vi "四点权值_白子.vi"(0 "3位置行":dbl, 1 "2位置行":dbl, 2 "1位置行":dbl, 3 "当前棋盘状态":i32[][](array[numeric]), 5 "4位置行":dbl, 9 "1位置列":i8, 11 "2位置列":i8, 12 "3位置列":i8, 13 "4位置列":i8) -> (4 "白子四位置权值":i32, 6 "有2个白子?或白子加无子?":bool, 8 "第1个是白子？":bool, 10 "3个白子?":bool, 14 "第一个位置为空？":bool, 15 "3个白子？或2个白子加无子":bool)   [LabVIEW 2018]
panel:
  out "第四位在框内？":bool
  out "第三位在框内？":bool
  out "第二位在框内？":bool
  out "第一位在框内？":bool
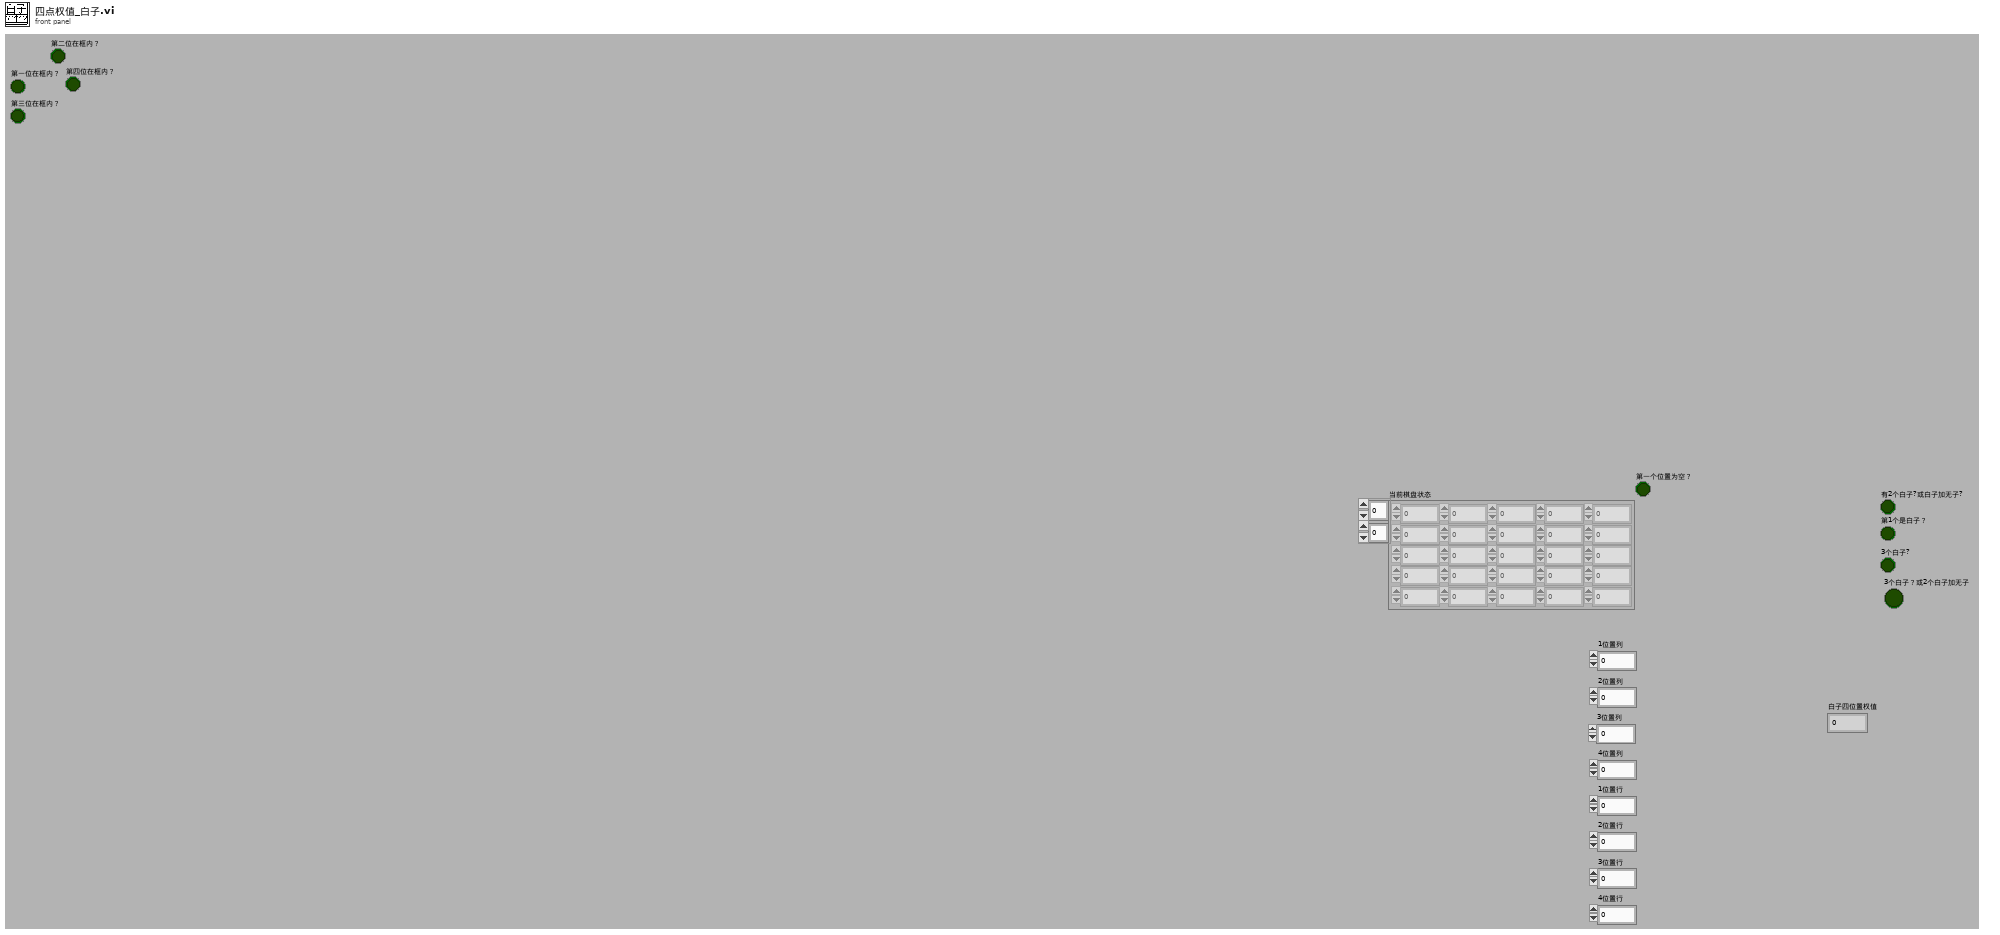
[diagram p1: front panel]
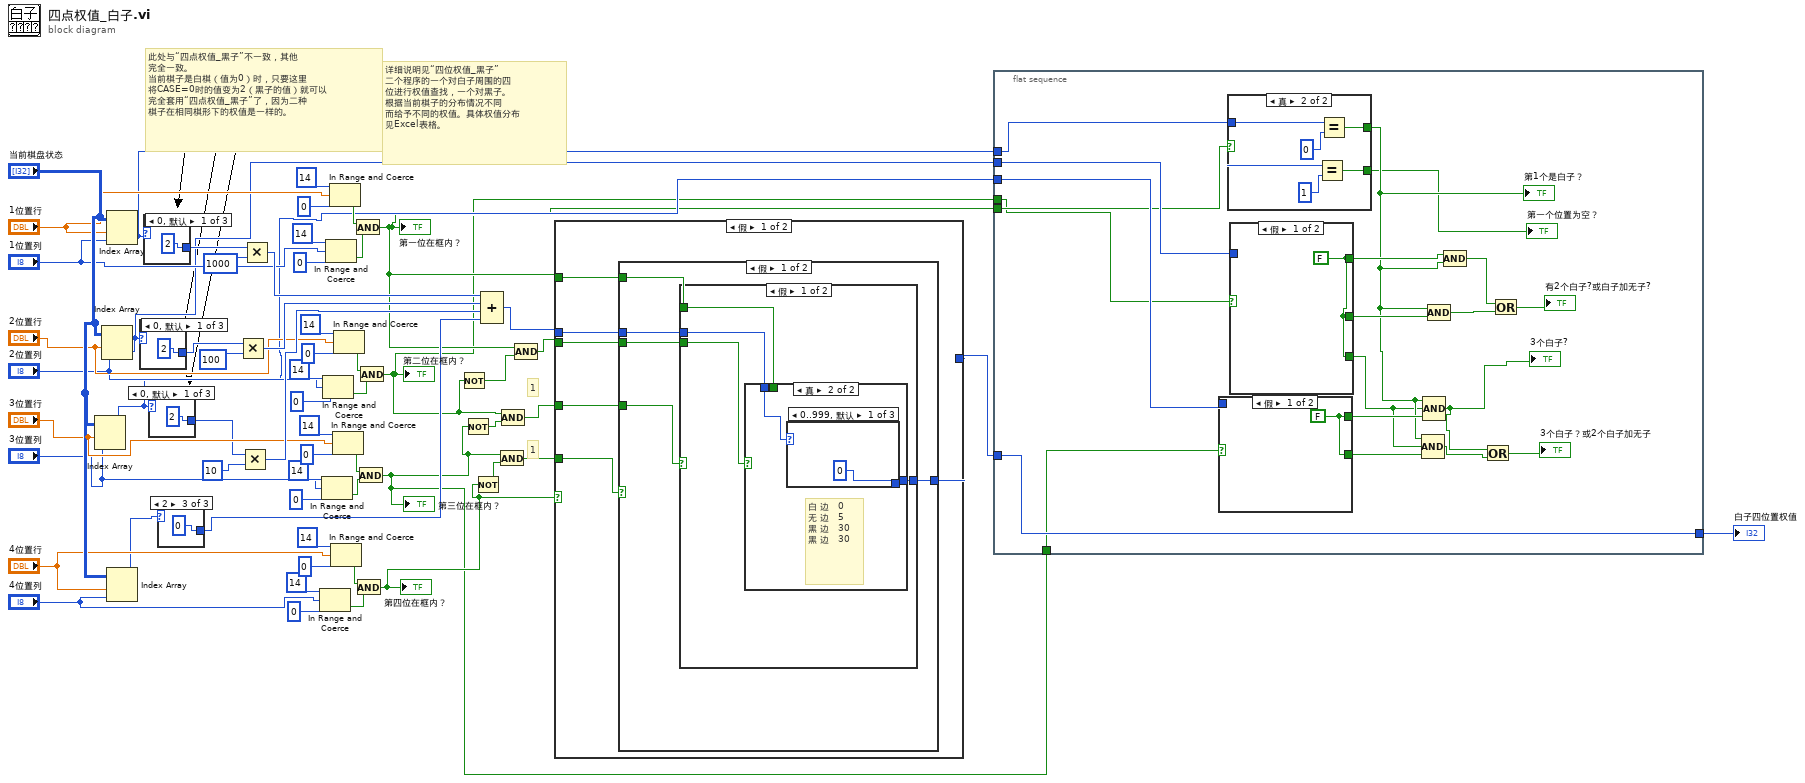
[diagram p0: block diagram]
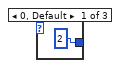
[diagram p2: hidden frame]
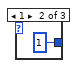
[diagram p3: hidden frame]
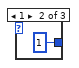
[diagram p4: hidden frame]
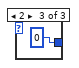
[diagram p5: hidden frame]
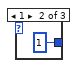
[diagram p6: hidden frame]
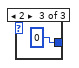
[diagram p7: hidden frame]
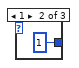
[diagram p8: hidden frame]
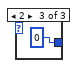
[diagram p9: hidden frame]
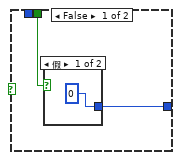
[diagram p10: hidden frame]
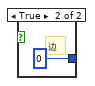
[diagram p11: hidden frame]
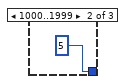
[diagram p12: hidden frame]
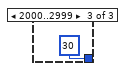
[diagram p13: hidden frame]
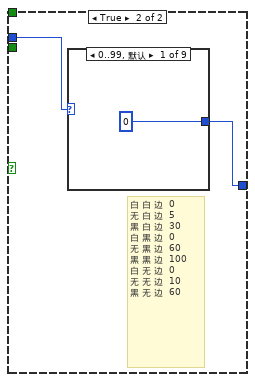
[diagram p14: hidden frame]
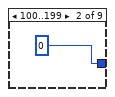
[diagram p15: hidden frame]
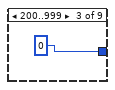
[diagram p16: hidden frame]
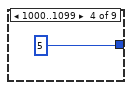
[diagram p17: hidden frame]
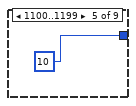
[diagram p18: hidden frame]
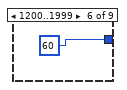
[diagram p19: hidden frame]
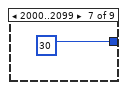
[diagram p20: hidden frame]
diagram:
  # "此处与“四点权值_黑子”不一致，其他\n完全一致。\n当前棋子是白棋（值为0）时，只要这里\n将CASE=0时的值变为2（黑子的值）就可以\n完全套用“四点权值_黑子”了，因为二种\n棋子在相同棋形下的权值是一样的。"
  # "详细说明见“四位权值_黑子”\n二个程序的一个对白子周围的四\n位进行权值查找，一个对黑子。\n根据当前棋子的分布情况不同\n而给予不同的权值。具体权值分布\n见Excel表格。"
  # "1"
  # "1"
  n1 = Index Array(array="当前棋盘状态", index (row)="3位置行", index (col)="3位置列") -> (element=w4:i32)
  n2 = Index Array(array="当前棋盘状态", index (row)="2位置行", index (col)="2位置列") -> (element=w5:i32)
  n3 = Index Array(array="当前棋盘状态", index (row)="1位置行", index (col)="1位置列") -> (element=w6:i32)
  n4 = Index Array(array="当前棋盘状态", index (row)="4位置行", index (col)="4位置列") -> (element=w8:i32)
  n5 = case shown="0, 默认" w5 {
    tunnel: [2 1 0] -> w10
    frame 0, Default {
    }
    frame 1 {
    }
    frame 2 {
    }
  }
  n6 = case shown="0, 默认" w6 {
    tunnel: [2 1 0] -> w11
    frame 0, Default {
    }
    frame 1 {
    }
    frame 2 {
    }
  }
  n7 = case shown="0, 默认" w4 {
    tunnel: [2 1 0] -> w9
    frame 0, Default {
    }
    frame 1 {
    }
    frame 2 {
    }
  }
  n8 = case shown="2" w8 {
    tunnel: [2 1 0] -> w7
    frame 0, Default {
    }
    frame 1 {
    }
    frame 2 {
    }
  }
  n9 = Multiply(x=w10, y=100) -> (x*y=w25:i32)
  n10 = Multiply(x=w9, y=10) -> (x*y=w24:i32)
  n11 = Multiply(x=w11, y=1000) -> (x*y=w26:i32)
  n12 = In Range and Coerce(upper limit=14, x="4位置列", lower limit=0) -> (In Range?=w40:bool)  [unwired: 1 out]
  n13 = In Range and Coerce(upper limit=14, x="3位置列", lower limit=0) -> (In Range?=w34:bool)  [unwired: 1 out]
  n14 = In Range and Coerce(upper limit=14, x="2位置列", lower limit=0) -> (In Range?=w54:bool)  [unwired: 1 out]
  n15 = In Range and Coerce(upper limit=14, x="1位置列", lower limit=0) -> (In Range?=w55:bool)  [unwired: 1 out]
  n16 = In Range and Coerce(upper limit=14, x="1位置行", lower limit=0) -> (In Range?=w56:bool)  [unwired: 1 out]
  n17 = In Range and Coerce(upper limit=14, x="4位置行", lower limit=0) -> (In Range?=w41:bool)  [unwired: 1 out]
  n18 = In Range and Coerce(upper limit=14, x="3位置行", lower limit=0) -> (In Range?=w35:bool)  [unwired: 1 out]
  n19 = In Range and Coerce(upper limit=14, x="2位置行", lower limit=0) -> (In Range?=w53:bool)  [unwired: 1 out]
  n20 = And(x=w56, y=w55) -> (x .and. y?=w3:bool)
  "第一位在框内？" <- w3
  n21 = And(x=w41, y=w40) -> (x .and. y?=w32:bool)
  "第四位在框内？" <- w32
  n22 = And(x=w35, y=w34) -> (x .and. y?=w1:bool)
  "第三位在框内？" <- w1
  n23 = And(x=w53, y=w54) -> (x .and. y?=w2:bool)
  "第二位在框内？" <- w2
  n24 = Not(x=w2) -> (.not. x?=w30:bool)
  n25 = Not(x=w1) -> (.not. x?=w28:bool)
  n26 = Not(x=w32) -> (.not. x?=w29:bool)
  n27 = Compound Arithmetic op=ADD(w26, w25, w24, w7) -> (w23:i32)
  n28 = And(x=w1, y=w29) -> (x .and. y?=w33:bool)
  n29 = Compound Arithmetic op=AND(w2, w28) -> (w31:bool)
  n30 = Compound Arithmetic op=AND(w3, w30) -> (w27:bool)
  n31 = case shown="假" w32 {
    tunnel: [w74 w126] -> w12
    tunnel: w33 -> [w78 _]
    tunnel: w31 -> [w77 _]
    tunnel: w27 -> [w76 _]
    tunnel: w3 -> [w75 _]
    tunnel: w23 -> [w73 w127]
    frame False {
      n32 = case shown="假" w78 {
        tunnel: w77 -> [w83 _]
        tunnel: w76 -> [w82 _]
        tunnel: w75 -> [w81 _]
        tunnel: [w80 w108] -> w74
        tunnel: w73 -> [w79 w109]
        frame False {
          n33 = case shown="假" w83 {
            tunnel: w82 -> [w87 _]
            tunnel: w81 -> [w86 _]
            tunnel: [w85 w97] -> w80
            tunnel: w79 -> [w84 w98]
            frame False {
              n34 = case shown="真" w87 {
                tunnel: w86 -> [w89 _]
                tunnel: [w88 w92] -> w85
                tunnel: w84 -> [_ w93]
                frame False {
                  n35 = case shown="假" w89 {
                    tunnel: [0 0] -> w88
                    frame False {
                    }
                    frame True {
                      # "边"
                    }
                  }
                }
                frame True {
                  # "白\t边\t\t\t0\n无\t边\t\t\t5\n黑\t边\t\t\t30\n黑\t边\t\t\t30"
                  n36 = case shown="0..999, 默认" w93 {
                    tunnel: [0 5 30] -> w92
                    frame 0..999, Default {
                    }
                    frame 1000..1999 {
                    }
                    frame 2000..2999 {
                    }
                  }
                }
              }
            }
            frame True {
              # "白\t白\t边\t\t0\n无\t白\t边\t\t5\n黑\t白\t边\t\t30\n白\t黑\t边\t\t0\n无\t黑\t边\t\t60\n黑\t黑\t边\t\t100\n白\t无\t边\t\t0\n无\t无\t边\t\t10\n黑\t无\t边\t\t60"
              n37 = case shown="0..99, 默认" w98 {
                tunnel: [0 0 0 5 10 60 30 60 100] -> w97
                frame 0..99, Default {
                }
                frame 100..199 {
                }
                frame 200..999 {
                }
                frame 1000..1099 {
                }
                frame 1100..1199 {
                }
                frame 1200..1999 {
                }
                frame 2000..2099 {
                }
                frame 2100..2199 {
                }
                frame 2200..2299 {
                }
              }
            }
          }
        }
        frame True {
          # "白\t白\t白\t边\t0\n无\t白\t白\t边\t5\n黑\t白\t白\t边\t30\n白\t黑\t白\t边\t0\n无\t黑\t白\t边\t60\n黑\t黑\t白\t边\t100\n白\t无\t白\t边\t0\n无\t无\t白\t边\t10\n黑\t无\t白\t边\t60\n白\t白\t黑\t边\t0\n无\t白\t黑\t边\t5\n黑\t白\t黑\t边\t30\n白\t黑\t黑\t边\t0\n无\t黑\t黑\t边\t600\n黑\t黑\t黑\t边\t2000\n白\t无\t黑\t边\t0\n无\t无\t黑\t边\t30\n黑\t无\t黑\t边\t800\n白\t白\t无\t边\t0\n无\t白\t无\t边\t5\n黑\t白\t无\t边\t30\n白\t黑\t无\t边\t0\n无\t黑\t无\t边\t100\n黑\t黑\t无\t边\t800\n白\t无\t无\t边\t0\n无\t无\t无\t边\t10\n黑\t无\t无\t边\t300"
          n38 = case shown="0..999, 默认" w109 {
            tunnel: [0 5 10 30 60 100 600 30 60 300 800 100 800 2000] -> w108
            frame 0..999, Default {
            }
            frame 1000..1029 {
            }
            frame 1100..1119 {
            }
            frame 1120..1129 {
            }
            frame 1200..1209 {
            }
            frame 1210..1219 {
            }
            frame 1220..1229 {
            }
            frame 2000..2029 {
            }
            frame 2100..2109 {
            }
            frame 2110..2119 {
            }
            frame 2120..2129 {
            }
            frame 2200..2209 {
            }
            frame 2210..2219 {
            }
            frame 2220 {
            }
          }
        }
      }
    }
    frame True {
      # "第四个仍在框内"
      # "无\t黑\t黑\t白\t600\n黑\t黑\t黑\t白\t2000\n无\t无\t黑\t白\t30\n黑\t无\t黑\t白\t800\n无\t黑\t无\t白\t100\n黑\t黑\t无\t白\t800\n无\t无\t无\t白\t10\n黑\t无\t无\t白\t300"
      # "无\t黑\t黑\t黑\t50000\n黑\t黑\t黑\t黑\t1000000\n无\t无\t黑\t黑\t2000\n黑\t无\t黑\t黑\t50000\n无\t黑\t无\t黑\t2000\n黑\t黑\t无\t黑\t50000\n无\t无\t无\t黑\t400\n黑\t无\t无\t黑\t2000\n无\t黑\t黑\t无\t5000\n黑\t黑\t黑\t无\t100000\n无\t无\t黑\t无\t600\n黑\t无\t黑\t无\t5000\n无\t黑\t无\t无\t8000\n黑\t黑\t无\t无\t10000\n无\t无\t无\t无\t100\n黑\t无\t无\t无\t1000"
      n39 = case shown="2121" w127 {
        tunnel: [5 5 10 100 400 10 30 600 2000 30 10 60 100 800 2000 100 600 5000 5000 600 60 5 30 60 300 1000 2000 300 800 5000 50000 800 60 100 800 10000 50000 800 2000 100000 1000000 2000 100 30 0 0] -> w125
        frame 1000..1099 {
        }
        frame 1100..1109 {
        }
        frame 1110 {
        }
        frame 1111 {
        }
        frame 1112 {
        }
        frame 1113 {
        }
        frame 1120 {
        }
        frame 1121 {
        }
        frame 1122 {
        }
        frame 1123 {
        }
        frame 1130..1139 {
        }
        frame 1200..1209 {
        }
        frame 1210 {
        }
        frame 1211 {
        }
        frame 1212 {
        }
        frame 1213 {
        }
        frame 1220 {
        }
        frame 1221 {
        }
        frame 1222 {
        }
        frame 1223 {
        }
        frame 1230..1239 {
        }
        frame 1300..1399 {
        }
        frame 2000..2099 {
        }
        frame 2100..2109 {
        }
        frame 2110 {
        }
        frame 2111 {
        }
        frame 2112 {
        }
        frame 2113 {
        }
        frame 2120 {
        }
        frame 2121 {
        }
        frame 2122 {
        }
        frame 2123 {
        }
        frame 2130..2139 {
        }
        frame 2200..2209 {
        }
        frame 2210 {
        }
        frame 2211 {
        }
        frame 2212 {
        }
        frame 2213 {
        }
        frame 2220 {
        }
        frame 2221 {
        }
        frame 2222 {
        }
        frame 2223 {
        }
        frame 2230..2239 {
        }
        frame 2300..2399 {
        }
        frame 3000..3999 {
        }
        frame 0..999, Default {
        }
      }
      n40 = Add(x=w125, y=100) -> (x+y=w126:i32)
    }
  }
  n41 = flat-sequence {
    tunnel: w6 -> [w179]
    tunnel: w5 -> [w178]
    tunnel: w4 -> [w177]
    tunnel: w12 -> [w180]
    tunnel: [w180] -> w13
    tunnel: w3 -> [w176]
    tunnel: w2 -> [w175]
    tunnel: w1 -> [w174]
    frame #0 {
      n42 = case shown="假" w174 {
        tunnel: [w194 w198] -> w193
        tunnel: [w194 w196] -> w185
        tunnel: w177 -> [_ w195]
        frame False {
          w194 = FALSE
        }
        frame True {
          n43 = Equal?(x=w195, y=1) -> (x = y?=w196:bool)
          n44 = Equal?(x=w195, y=0) -> (x = y?=w198:bool)
        }
      }
      n45 = case shown="真" w176 {
        tunnel: [w208 w212] -> w184
        tunnel: [w208 w210] -> w182
        tunnel: w179 -> [_ w209]
        frame False {
          w208 = FALSE
        }
        frame True {
          n46 = Equal?(x=w209, y=1) -> (x = y?=w210:bool)
          n47 = Equal?(x=w209, y=0) -> (x = y?=w212:bool)
        }
      }
      "第1个是白子？" <- w184
      "第一个位置为空？" <- w182
      n48 = case shown="假" w175 {
        tunnel: [w200 w205] -> w192
        tunnel: [w200 w203] -> w191
        tunnel: [w200 w202] -> w183
        tunnel: w178 -> [_ w201]
        frame False {
          w200 = FALSE
        }
        frame True {
          n49 = Equal?(x=w201, y=0) -> (x = y?=w202:bool)
          n50 = Equal?(x=w201, y=1) -> (x = y?=w205:bool)
          n51 = Equal?(x=w201, y=0) -> (x = y?=w203:bool)
        }
      }
      n52 = Compound Arithmetic op=AND(w184, w183, w185) -> (w187:bool)
      n53 = Compound Arithmetic op=AND(w184, w183, w193) -> (w181:bool)
      "3个白子?" <- w181
      n54 = Compound Arithmetic op=AND(w184, w192) -> (w189:bool)
      n55 = Compound Arithmetic op=AND(w191, w184) -> (w190:bool)
      n56 = Or(x=w181, y=w187) -> (x .or. y?=→"3个白子？或2个白子加无子":bool)
      n57 = Or(x=w190, y=w189) -> (x .or. y?=→"有2个白子?或白子加无子?":bool)
    }
  }
  "白子四位置权值" <- w13
